vi "OPEN PORT-CLOSE PORT(SubVI).vi"(8 "error in (no error)":errorcluster, 10 "Enum":enum16{"OPEN PORT", "CLOSE PORT"}(ring), 11 "VISA Refnum in":refnum<visa-resource-name>) -> (0 "error out":errorcluster, 3 "VISA Refnum out":refnum<visa-resource-name>)   [LabVIEW 2014, in "CAP-USB.lvlib"]
doc: "Este VI se encarga de abrir el puerto o cerrarlo dependiendo\ndel comando que se le ingrese"
uses:
  CAP-USB.lvlib
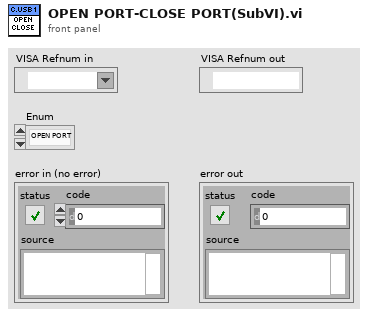
[diagram p1: front panel]
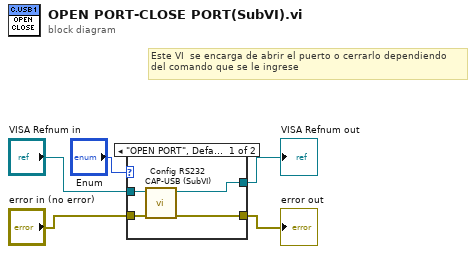
[diagram p0: block diagram]
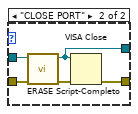
[diagram p2: hidden frame]
diagram:
  # "Este VI  se encarga de abrir el puerto o cerrarlo dependiendo\ndel comando que se le ingrese"
  n1 = case shown="\"OPEN PORT\", Default" "Enum" {
    tunnel: "VISA Refnum in" -> [w9 w10]
    tunnel: "error in (no error)" -> [w8 w11]
    tunnel: [w7 w13] -> w3
    tunnel: [w6 w14] -> w4
    frame "OPEN PORT", Default {
      n2 = call "Config RS232 CAP-USB (SubVI).vi"("error in (no error)"=w8, "VISA Refnum in"=w9) -> ("error out"=w6:errorcluster, "VISA Refnum out"=w7:refnum<visa-resource-name>)  [unwired: 8 in]
    }
    frame "CLOSE PORT" {
      n3 = call "ERASE Script-Completo.vi"("error in (no error)"=w11, "VISA resource name"=w10) -> ("error out"=w12:errorcluster, "VISA resource name out"=w13:refnum<visa-resource-name>)  [unwired: 8 in]
      n4 = VISA Close(VISA resource name=w13, error in (no error)=w12) -> (error out=w14:errorcluster)
    }
  }
  "error out" <- w4
  "VISA Refnum out" <- w3
